vi "Circle Area Perimeter.vi"() -> ()   [LabVIEW 2021]
panel:
  out "perimeter":dbl
  out "area":dbl
  in  "r":dbl
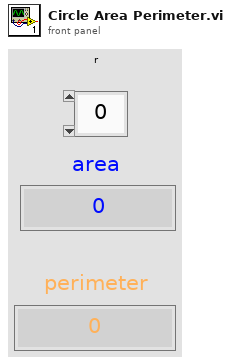
[diagram p1: front panel]
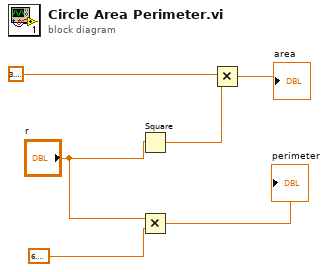
[diagram p0: block diagram]
diagram:
  n1 = Square(x="r") -> (x^2=w5:dbl)
  n2 = Multiply(x="r", y=6.283185307179586) -> (x*y=→"perimeter":dbl)
  n3 = Multiply(x=w5, y=3.141592653589793) -> (x*y=→"area":dbl)
